vi "OPCWrite.vi"(1 "Data to Write":i32[](array[numeric])=[0, 0, 0, 0, 0, 0], 2 "OPC URL":string) -> ()   [LabVIEW 2013]
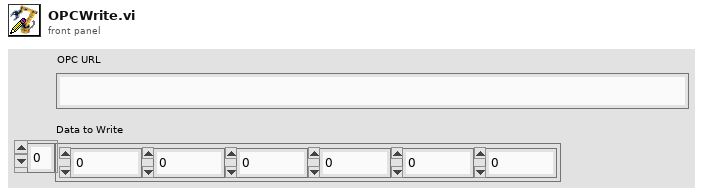
[diagram p1: front panel]
types:
  T1 = enum16{"Read", "Write", "ReadWrite", "BufferedRead", "BufferedReadWrite"}
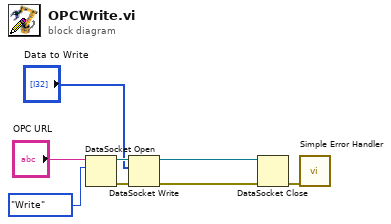
[diagram p0: block diagram]
diagram:
  n1 = DataSocket Open(10:T1."Write" ("mode"), 11:"OPC URL") -> (0:w6:errorcluster, 3:w8:refnum<k13>)  [unwired: 1 in, 1 out]
  n2 = DataSocket Write(8:w6, 10:"Data to Write", 11:w8) -> (0:w5:errorcluster, 3:w7:refnum<k13>)  [unwired: 1 in, 1 out]
  n3 = DataSocket Close(8:w5, 11:w7) -> (0:w4:errorcluster)  [unwired: 2 out]
  n4 = call <vilib>:"Simple Error Handler.vi"("error in (no error)"=w4) -> ()  [unwired: 4 in, 5 out]
